vi "SmartSEM Remote API get FIB HV data.vi"(8 "error in":errorcluster, 11 "Api in":refnum<k7>(container)) -> (0 "error out":errorcluster, 1 "FIB parameters":T3 {"FIB probe current" format="%.3f"}, 2 "Capella HV Data Output":T1 {"Column Vac (Torr)" format="%.2e"; "Gun Vac (Torr)" format="%.2e"; "Lens2 Actual (V)" format="%.1f"; "Lens1 Actual (V)" format="%.1f"; "Emission Actual (uA)" format="%.3f"; "Extrator Actual (V)" format="%.2f"; "Tip Lifetime (uAhr)" format="%.2f"; "Lens2 Target (V)" format="%.1f"; "Lens1 Target (V)" format="%.1f"; "Faraday I (nA)" format="%.3f"; "Suppressor (V)" format="%.1f"; "Emission Target (uA)" format="%.3f"; "Extrator Target (V)" format="%.2f"; "Accelerator Actual (V)" format="%.2f"; "Accelerator Target (V)" format="%.2f"; "Filament (A)" format="%.2f"}, 3 "Api out":refnum<k7>)   [LabVIEW 2018]
panel:
  out "HV Data Output":T2 {"Tip Lifetime (hr)" format="%.2f"; "Lens2I (uA)" format="%.3f"; "Lens2 (V)" format="%.1f"; "Lens1I (uA)" format="%.3f"; "Lens1 (V)" format="%.1f"; "SuppI (uA)" format="%.3f"; "Suppressor (V)" format="%.1f"; "Emission (uA)" format="%.3f"; "Extrator (V)" format="%.1f"; "AccI (uA)" format="%.3f"; "Accelerator (V)" format="%.1f"; "Filament (A)" format="%.2f"}
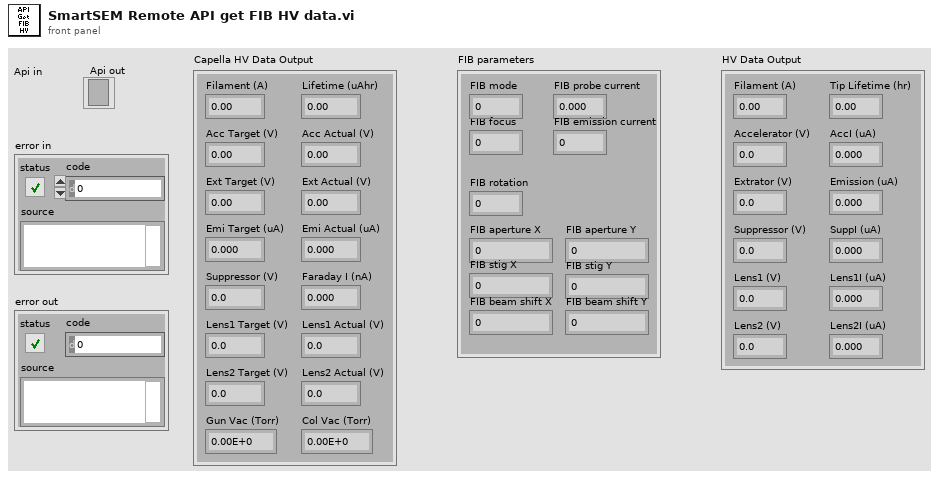
[diagram p1: front panel]
types:
  T1 = cluster{"Filament (A)":sgl, "Accelerator Target (V)":sgl, "Accelerator Actual (V)":sgl, "Extrator Target (V)":sgl, "Extrator Actual (V)":sgl, "Emission Target (uA)":sgl, "Emission Actual (uA)":sgl, "Suppressor (V)":sgl, "Faraday I (nA)":sgl, "Lens1 Target (V)":sgl, "Lens1 Actual (V)":sgl, "Lens2 Target (V)":sgl, "Lens2 Actual (V)":sgl, "Gun Vac (Torr)":sgl, "Column Vac (Torr)":sgl, "Tip Lifetime (uAhr)":sgl}
  T2 = cluster{"Filament (A)":sgl, "Accelerator (V)":sgl, "AccI (uA)":sgl, "Extrator (V)":sgl, "Emission (uA)":sgl, "Suppressor (V)":sgl, "SuppI (uA)":sgl, "Lens1 (V)":sgl, "Lens1I (uA)":sgl, "Lens2 (V)":sgl, "Lens2I (uA)":sgl, "Tip Lifetime (hr)":sgl}
  T3 = cluster{"FIB mode":u8, "FIB focus":sgl, "FIB probe current":sgl, "FIB emission current":sgl, "FIB rotation":sgl, "FIB aperture X":sgl, "FIB aperture Y":sgl, "FIB stig X":sgl, "FIB stig Y":sgl, "FIB beam shift X":sgl, "FIB beam shift Y":sgl}
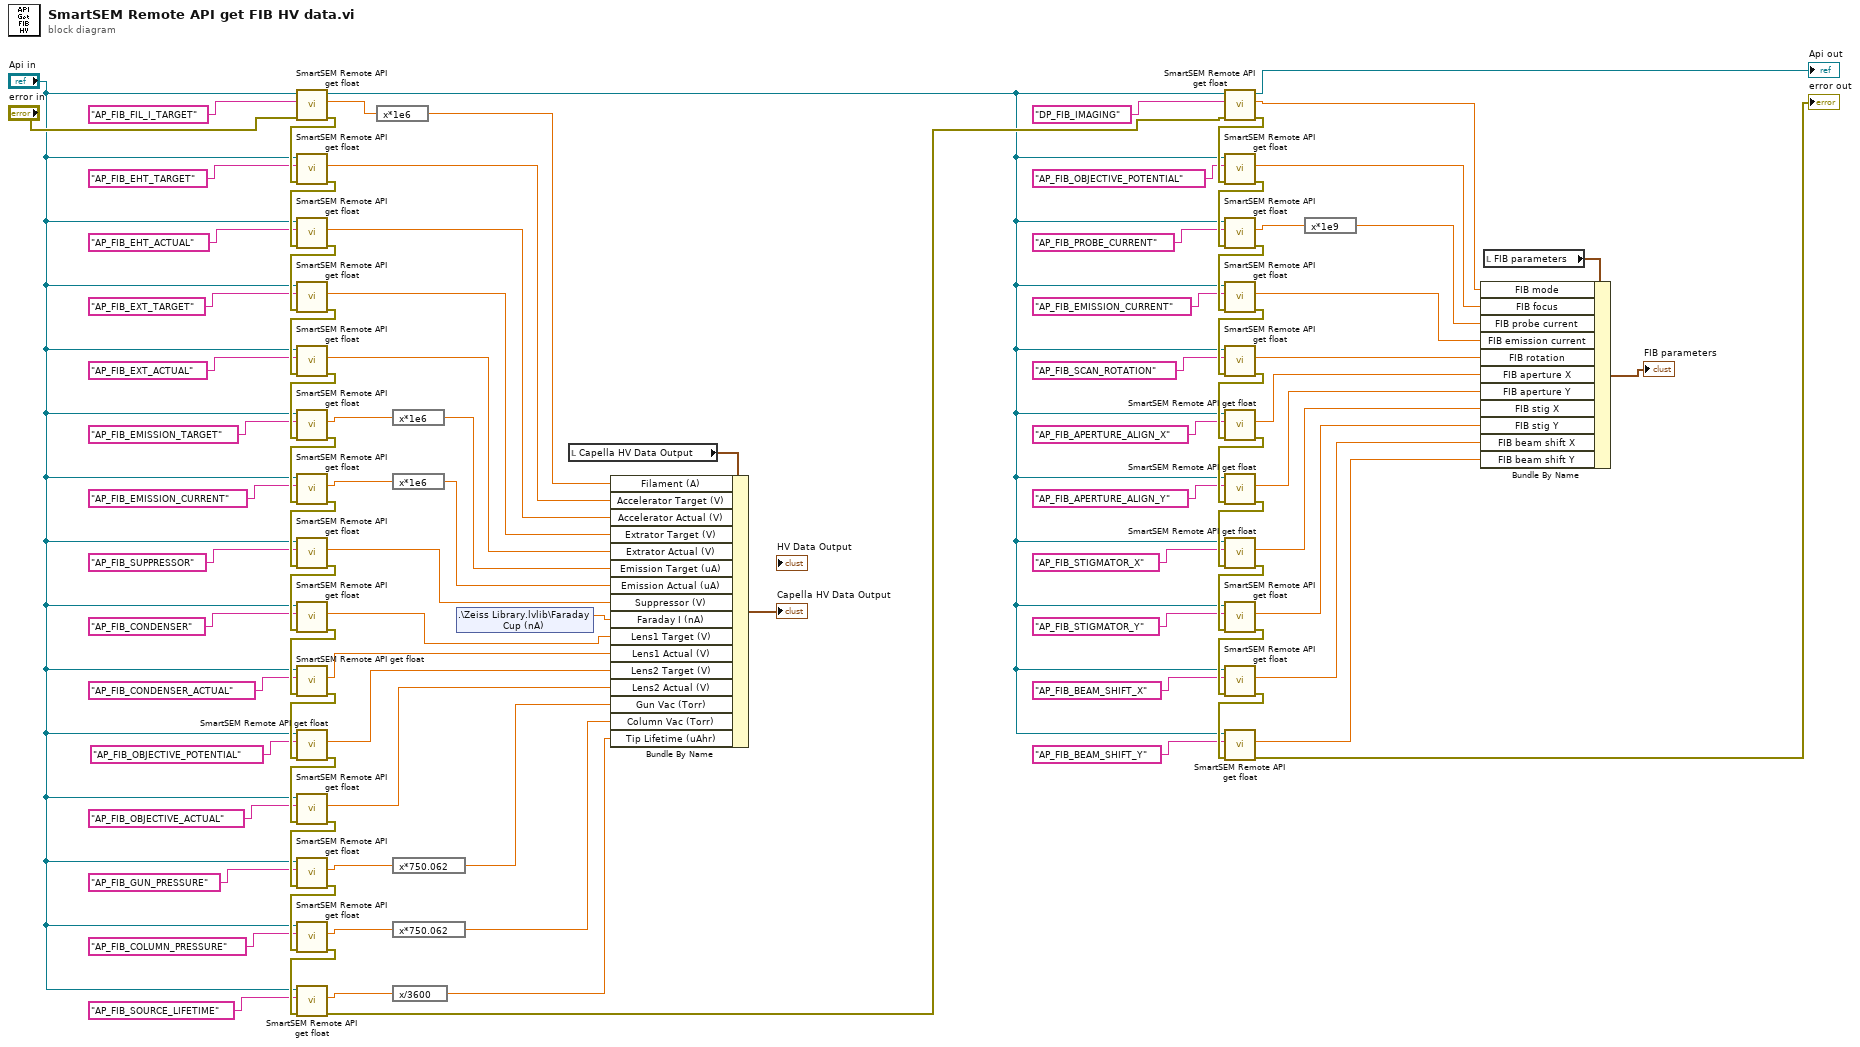
[diagram p0: block diagram]
diagram:
  n1 = call "SmartSEM Remote API get float.vi"("error in"="error in", "lpszParam"="AP_FIB_FIL_I_TARGET", "Api"="Api in") -> ("error out"=w79:errorcluster, "vValue"=w80:sgl, "Api out"=w1:refnum<k7>)  [unwired: 6 in]
  n2 = call "SmartSEM Remote API get float.vi"("error in"=w79, "lpszParam"="AP_FIB_EHT_TARGET", "Api"="Api in") -> ("error out"=w76:errorcluster, "vValue"=w77:sgl)  [unwired: 6 in, 1 out]
  n3 = call "SmartSEM Remote API get float.vi"("error in"=w76, "lpszParam"="AP_FIB_EHT_ACTUAL", "Api"="Api in") -> ("error out"=w73:errorcluster, "vValue"=w74:sgl)  [unwired: 6 in, 1 out]
  n4 = call "SmartSEM Remote API get float.vi"("error in"=w73, "lpszParam"="AP_FIB_EXT_TARGET", "Api"="Api in") -> ("error out"=w72:errorcluster, "vValue"=w70:sgl)  [unwired: 6 in, 1 out]
  n5 = call "SmartSEM Remote API get float.vi"("error in"=w72, "lpszParam"="AP_FIB_EXT_ACTUAL", "Api"="Api in") -> ("error out"=w71:errorcluster, "vValue"=w69:sgl)  [unwired: 6 in, 1 out]
  n6 = call "SmartSEM Remote API get float.vi"("error in"=w71, "lpszParam"="AP_FIB_EMISSION_TARGET", "Api"="Api in") -> ("error out"=w61:errorcluster, "vValue"=w60:sgl)  [unwired: 6 in, 1 out]
  n7 = call "SmartSEM Remote API get float.vi"("error in"=w61, "lpszParam"="AP_FIB_EMISSION_CURRENT", "Api"="Api in") -> ("error out"=w62:errorcluster, "vValue"=w59:sgl)  [unwired: 6 in, 1 out]
  n8 = call "SmartSEM Remote API get float.vi"("error in"=w62, "lpszParam"="AP_FIB_SUPPRESSOR", "Api"="Api in") -> ("error out"=w63:errorcluster, "vValue"=w51:sgl)  [unwired: 6 in, 1 out]
  n9 = call "SmartSEM Remote API get float.vi"("error in"=w63, "lpszParam"="AP_FIB_CONDENSER", "Api"="Api in") -> ("error out"=w64:errorcluster, "vValue"=w50:sgl)  [unwired: 6 in, 1 out]
  n10 = call "SmartSEM Remote API get float.vi"("error in"=w64, "lpszParam"="AP_FIB_CONDENSER_ACTUAL", "Api"="Api in") -> ("error out"=w65:errorcluster, "vValue"=w49:sgl)  [unwired: 6 in, 1 out]
  n11 = call "SmartSEM Remote API get float.vi"("error in"=w65, "lpszParam"="AP_FIB_OBJECTIVE_POTENTIAL", "Api"="Api in") -> ("error out"=w66:errorcluster, "vValue"=w41:sgl)  [unwired: 6 in, 1 out]
  n12 = call "SmartSEM Remote API get float.vi"("error in"=w66, "lpszParam"="AP_FIB_OBJECTIVE_ACTUAL", "Api"="Api in") -> ("error out"=w46:errorcluster, "vValue"=w40:sgl)  [unwired: 6 in, 1 out]
  n13 = call "SmartSEM Remote API get float.vi"("error in"=w46, "lpszParam"="AP_FIB_GUN_PRESSURE", "Api"="Api in") -> ("error out"=w48:errorcluster, "vValue"=w39:sgl)  [unwired: 6 in, 1 out]
  n14 = call "SmartSEM Remote API get float.vi"("error in"=w48, "lpszParam"="AP_FIB_COLUMN_PRESSURE", "Api"="Api in") -> ("error out"=w47:errorcluster, "vValue"=w38:sgl)  [unwired: 6 in, 1 out]
  n15 = call "SmartSEM Remote API get float.vi"("error in"=w47, "lpszParam"="AP_FIB_SOURCE_LIFETIME", "Api"="Api in") -> ("error out"=w26:errorcluster, "vValue"=w37:sgl)  [unwired: 6 in, 1 out]
  n16 = expression code="x*1e6"(w80) -> (w94:sgl)
  n17 = expression code="x*1e6"(w60) -> (w86:sgl)
  n18 = expression code="x*1e6"(w59) -> (w85:sgl)
  n19 = expression code="x*750.062"(w39) -> (w92:sgl)
  n20 = expression code="x*750.062"(w38) -> (w91:sgl)
  n21 = expression code="x/3600"(w37) -> (w89:sgl)
  n22 = shared-variable ".\\Zeiss Library.lvlib\\Faraday Cup (nA)"() -> (w83:sgl)  [unwired: 1 in, 1 out]
  n23 = local read "Capella HV Data Output"() -> (w93:T1)
  n24 = Bundle By Name(cluster=w93, "Filament (A)"=w94, "Accelerator Target (V)"=w77, "Accelerator Actual (V)"=w74, "Extrator Target (V)"=w70, "Extrator Actual (V)"=w69, "Emission Target (uA)"=w86, "Emission Actual (uA)"=w85, "Suppressor (V)"=w51, "Faraday I (nA)"=w83, "Lens1 Target (V)"=w50, "Lens1 Actual (V)"=w49, "Lens2 Target (V)"=w41, "Lens2 Actual (V)"=w40, "Gun Vac (Torr)"=w92, "Column Vac (Torr)"=w91, "Tip Lifetime (uAhr)"=w89) -> (→"Capella HV Data Output":T1)
  n25 = call "SmartSEM Remote API get float.vi"("error in"=w26, "lpszParam"="DP_FIB_IMAGING", "Api"=w1) -> ("error out"=w27:errorcluster, "vValue"=w11:sgl, "Api out"=→"Api out":refnum<k7>)  [unwired: 6 in]
  n26 = call "SmartSEM Remote API get float.vi"("error in"=w27, "lpszParam"="AP_FIB_OBJECTIVE_POTENTIAL", "Api"=w1) -> ("error out"=w28:errorcluster, "vValue"=w10:sgl)  [unwired: 6 in, 1 out]
  n27 = call "SmartSEM Remote API get float.vi"("error in"=w28, "lpszParam"="AP_FIB_PROBE_CURRENT", "Api"=w1) -> ("error out"=w29:errorcluster, "vValue"=w12:sgl)  [unwired: 6 in, 1 out]
  n28 = call "SmartSEM Remote API get float.vi"("error in"=w29, "lpszParam"="AP_FIB_EMISSION_CURRENT", "Api"=w1) -> ("error out"=w30:errorcluster, "vValue"=w9:sgl)  [unwired: 6 in, 1 out]
  n29 = call "SmartSEM Remote API get float.vi"("error in"=w30, "lpszParam"="AP_FIB_SCAN_ROTATION", "Api"=w1) -> ("error out"=w31:errorcluster, "vValue"=w8:sgl)  [unwired: 6 in, 1 out]
  n30 = call "SmartSEM Remote API get float.vi"("error in"=w31, "lpszParam"="AP_FIB_APERTURE_ALIGN_X", "Api"=w1) -> ("error out"=w36:errorcluster, "vValue"=w7:sgl)  [unwired: 6 in, 1 out]
  n31 = call "SmartSEM Remote API get float.vi"("error in"=w36, "lpszParam"="AP_FIB_APERTURE_ALIGN_Y", "Api"=w1) -> ("error out"=w35:errorcluster, "vValue"=w6:sgl)  [unwired: 6 in, 1 out]
  n32 = call "SmartSEM Remote API get float.vi"("error in"=w35, "lpszParam"="AP_FIB_STIGMATOR_X", "Api"=w1) -> ("error out"=w34:errorcluster, "vValue"=w5:sgl)  [unwired: 6 in, 1 out]
  n33 = call "SmartSEM Remote API get float.vi"("error in"=w34, "lpszParam"="AP_FIB_STIGMATOR_Y", "Api"=w1) -> ("error out"=w33:errorcluster, "vValue"=w4:sgl)  [unwired: 6 in, 1 out]
  n34 = call "SmartSEM Remote API get float.vi"("error in"=w33, "lpszParam"="AP_FIB_BEAM_SHIFT_X", "Api"=w1) -> ("error out"=w32:errorcluster, "vValue"=w3:sgl)  [unwired: 6 in, 1 out]
  n35 = call "SmartSEM Remote API get float.vi"("error in"=w32, "lpszParam"="AP_FIB_BEAM_SHIFT_Y", "Api"=w1) -> ("error out"=→"error out":errorcluster, "vValue"=w2:sgl)  [unwired: 6 in, 1 out]
  n36 = expression code="x*1e9"(w12) -> (w84:sgl)
  n37 = local read "FIB parameters"() -> (w88:T3)
  n38 = Bundle By Name(cluster=w88, "FIB mode"=w11, "FIB focus"=w10, "FIB probe current"=w84, "FIB emission current"=w9, "FIB rotation"=w8, "FIB aperture X"=w7, "FIB aperture Y"=w6, "FIB stig X"=w5, "FIB stig Y"=w4, "FIB beam shift X"=w3, "FIB beam shift Y"=w2) -> (→"FIB parameters":T3)
